vi "Query Available Signal Paths.vi"(8 "error in (no error)":errorcluster, 10 "Instance (1)":i32=1, 11 "VISA resource name":refnum<visa-resource-name>) -> (0 "error out":errorcluster, 2 "Available Signal Paths":string, 3 "VISA resource name out":refnum<visa-resource-name>)   [LabVIEW 2020, in "Rohde&Schwarz CMXP GPRF.lvlib"]
doc: "Returns the names of the available signal paths.\n\nAttribute(s):\nRSCMXPGPRF_ATTR_AVAILABLE_SIGNAL_PATHS\n\nRemote-control command(s):\nCATalog:GPRF:MEAS<i>:SPATh<stream>?"
uses:
  <instrlib>/Rohde&Schwarz CMXP GPRF/Rohde&Schwarz CMXP GPRF.lvlib
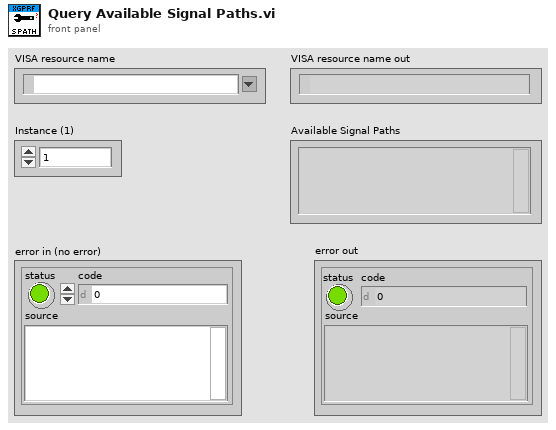
[diagram p1: front panel]
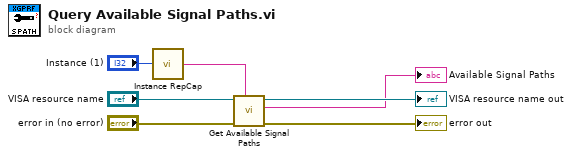
[diagram p0: block diagram]
diagram:
  n1 = call <instrlib>:"Instance RepCap.vi"("Instance in"="Instance (1)") -> ("Instance out"=w3:string)
  n2 = call "Get Available Signal Paths"("Repeated Capabilities"=w3, "error in (no error)"="error in (no error)", "instrument handle"="VISA resource name") -> ("error out"=→"error out":errorcluster, "Available Signal Paths"=→"Available Signal Paths":string, "instrument handle out"=→"VISA resource name out":refnum<visa-resource-name>)  [unwired: 6 in]
